vi "Read connection counter.vi"(8 "error in (no error)":errorcluster, 11 "TCP slave in":refnum<class "TCP Slave.lvclass">) -> (0 "error out":errorcluster, 2 "currently connected":u32, 3 "TCP slave out":refnum<class "TCP Slave.lvclass">)   [LabVIEW 2020, in "SubVIs.lvlib" / "TCP Slave.lvclass"]
uses:
  <vilib>/Modbus/subvis/Protocol/TCP/TCP Slave/TCP Slave.lvclass
  <vilib>/Modbus/subvis/Protocol/TCP/TCP Slave/TCP Slave.lvclass/TCP Slave.ctl
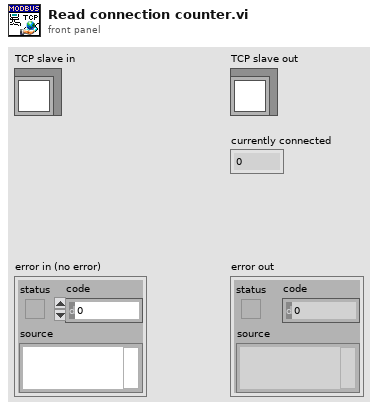
[diagram p1: front panel]
types:
  T1 = typedef "SubVIs.lvlib/TCP Slave.lvclass/Connection Counter.ctl" = cluster{"Currently Connected":u32, "Connection Records":refnum<data-value>[]}
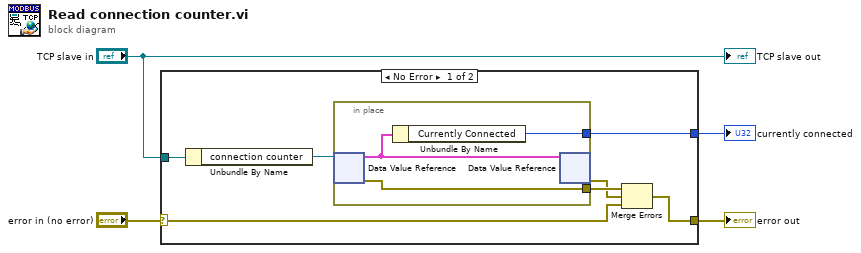
[diagram p0: block diagram]
diagram:
  n1 = case shown="No Error" "error in (no error)" {
    selector: "error in (no error)" -> [w6 w15]
    tunnel: "TCP slave in" -> [w11 _]
    tunnel: [w10 w15] -> w3
    tunnel: [w8 _] -> w2
    frame No Error {
      n2 = Unbundle By Name(w11) -> ("connection counter"=w9:refnum<data-value>)
      n3 = in-place {
        in-place-border: [w13] -> w8
        in-place-border: [w12] -> w7
        n4 = in-place-dvr #1(w9) -> (w14:T1, w12:errorcluster)
        n5 = Unbundle By Name(w14) -> ("Currently Connected"=w13:u32)
        n6 = in-place-dvr #1(w14) -> (w5:errorcluster)  [unwired: 1 out]
      }
      n7 = Merge Errors(w7, w5, w6) -> (w10:errorcluster)
    }
    frame Error {
    }
  }
  "error out" <- w3
  "currently connected" <- w2
  "TCP slave out" <- "TCP slave in"
